vi "UpdateConfiguration.vi"(2 "error in (no error)":errorcluster, 3 "ConfigIn":T1={"IntTime"=100, "Samples"=3, "PowerMin"=300.0, "KneeMin"=-20.0, "KneeMax"=20.0} {"IntTime" min=1 max=100000; "PowerMin" min=0.0 max=10000.0; "KneeMin" min=-40.0 max=0.0; "KneeMax" min=0.0 max=40.0; "Samples" min=1 max=10}, 4 "Instruments in":refnum<class "Instruments.lvclass">) -> (0 "error out":errorcluster, 1 "Instruments out":refnum<class "Instruments.lvclass">)   [LabVIEW 2012, in "Instruments.lvclass"]
uses:
  Instruments.lvclass
  Controls/Config.ctl
  Instruments.lvclass/Instruments.ctl
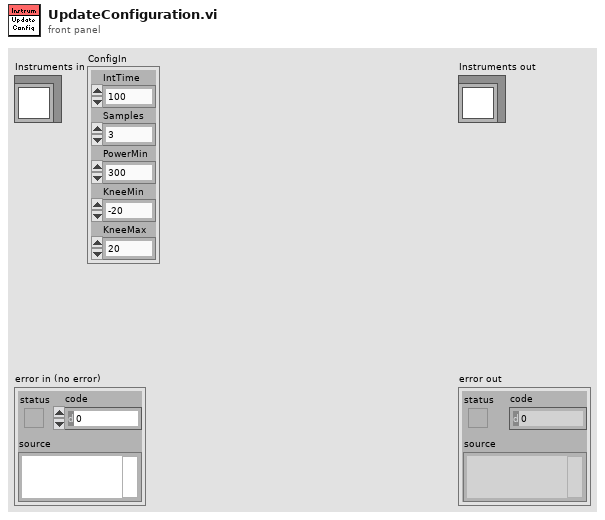
[diagram p1: front panel]
types:
  T1 = typedef "Config.ctl" = cluster{"IntTime":i32, "Samples":i32, "PowerMin":dbl, "KneeMin":dbl, "KneeMax":dbl}
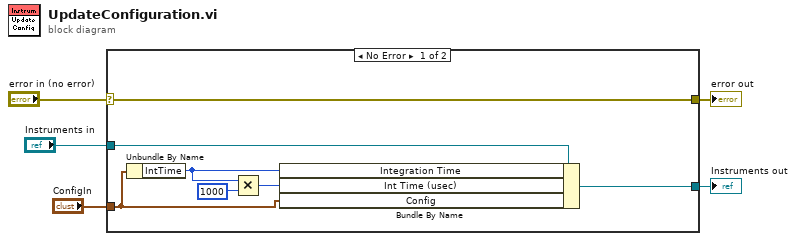
[diagram p0: block diagram]
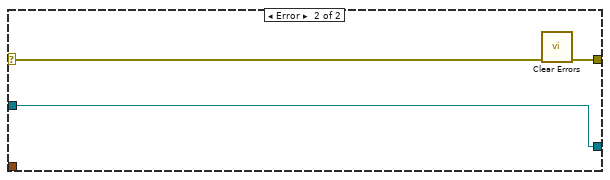
[diagram p2: hidden frame]
diagram:
  n1 = case shown="No Error" "error in (no error)" {
    selector: "error in (no error)" -> [w6 w14]
    tunnel: [w6 w13] -> w4
    tunnel: [w7 w15] -> w2
    tunnel: "Instruments in" -> [w12 w15]
    tunnel: "ConfigIn" -> [w8 _]
    frame No Error {
      n2 = Unbundle By Name(w8) -> ("IntTime"=w10:i32)
      n3 = Multiply(x=w10, y=1000) -> (x*y=w9:i32)
      n4 = Bundle By Name(cluster=w12, "Integration Time"=w10, "Int Time (usec)"=w9, "Config"=w8) -> (w7:refnum<class "Instruments.lvclass">)
    }
    frame Error {
      n5 = call <vilib>:"Clear Errors.vi"("error in (no error)"=w14) -> ("error out"=w13:errorcluster)  [unwired: 6 in]
    }
  }
  "error out" <- w4
  "Instruments out" <- w2
